vi "save data.vi"(8 "backwashing?":bool, 9 "coagulant dose":dbl) -> ()   [LabVIEW 2015]
uses:
  Sensor buffer command.ctl
panel:
  out "data labels":string[](array[string])
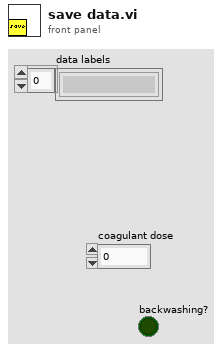
[diagram p1: front panel]
types:
  T1 = typedef "Sensor buffer command.ctl" = enum16{"set buffer size", "write", "refill buffer", "read recent", "read all", "clear"}
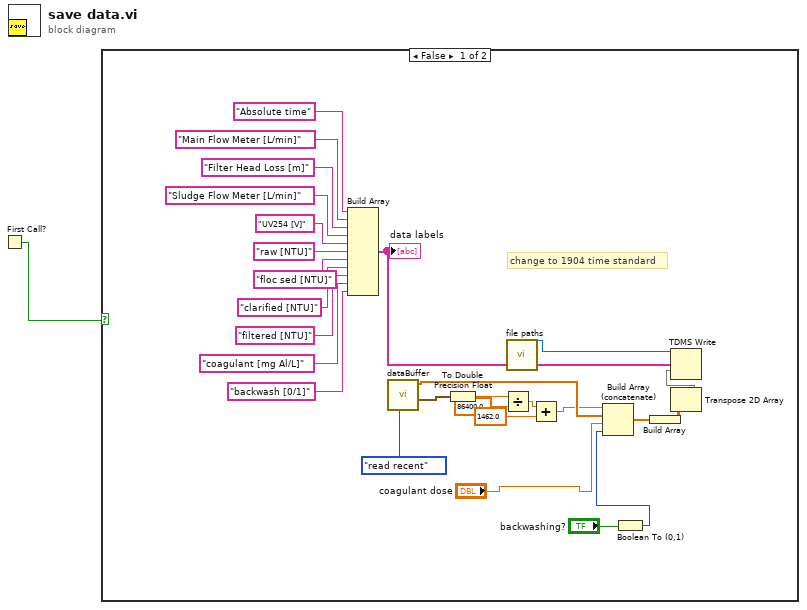
[diagram p0: block diagram]
diagram:
  n1 = First Call?() -> (First Call?: T/F=w1:bool)
  n2 = case shown="False" w1 {
    frame False {
      # "change to 1904 time standard"
      n3 = Build Array("Absolute time", "Main Flow Meter [L/min]", "Filter Head Loss [m]", "Sludge Flow Meter [L/min]", "UV254 [V]" ("element"), "raw [NTU]", "floc sed [NTU]", "clarified [NTU]", "filtered [NTU]" ("element"), "coagulant [mg Al/L]" ("element"), "backwash [0/1]" ("element")) -> (w15:string[])
      "data labels" <- w15
      n4 = call "dataBuffer.vi"("command"=Sensor_buffer_command."read recent") -> ("recent time"=w11:timestamp, "recent data"=w14:dbl[])  [unwired: 5 in, 4 out]
      n5 = To Double Precision Float(number=w11) -> (double precision float=w6:dbl)
      n6 = Divide(x=w6, y=86400.0) -> (x/y=w4:dbl)
      n7 = call "file paths.vi"() -> ("datalog"=w28:refnum<k34>)  [unwired: 8 in, 3 out]
      n8 = Add(x=w4, y=1462.0) -> (x+y=w2:dbl)
      n9 = Boolean To (0,1)(Boolean="backwashing?") -> (0, 1=w12:i16)
      n10 = Build Array (concatenate)(w2, w14, "coagulant dose", w12) -> (w10:dbl[])
      n11 = Build Array(w10) -> (w8:dbl[][])
      n12 = Transpose 2D Array(2D array=w8) -> (transposed array=w7:dbl[][])
      n13 = TDMS Write(0:w28, 7:w15, 9:w7) -> ()  [unwired: 3 in, 4 out]
    }
    frame True {
    }
  }
